vi "PFI-28000-System_Get Channels Per Card.vi"(8 "error in (no error)":errorcluster, 11 "PFI-28000-System in":refnum<class "PFI-28000-System.lvclass">) -> (0 "error out":errorcluster, 2 "Channels Per Card":i32, 3 "PFI-28000-System out":refnum<class "PFI-28000-System.lvclass">)   [LabVIEW 2017, in "PFI-28000-System.lvclass"]
uses:
  PFI-28000-System.lvclass
  Utilities/PFI-28000-Utils.lvlib
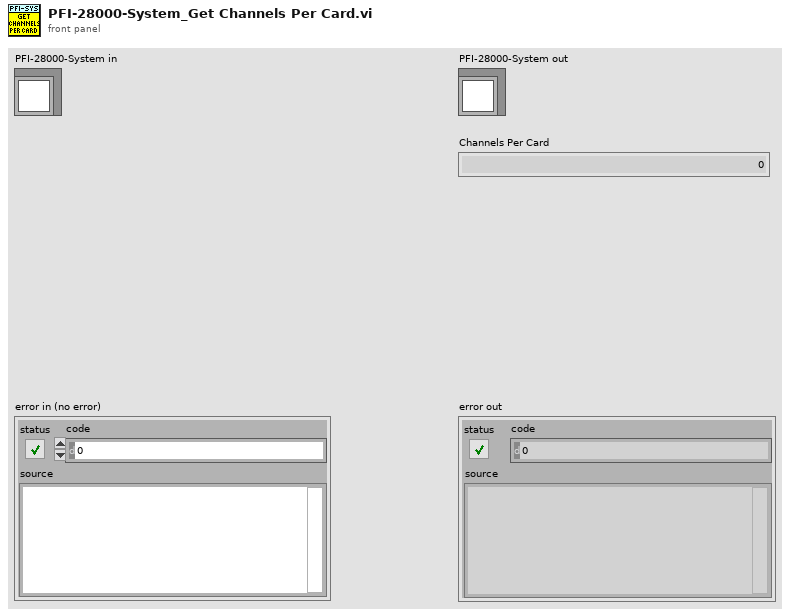
[diagram p1: front panel]
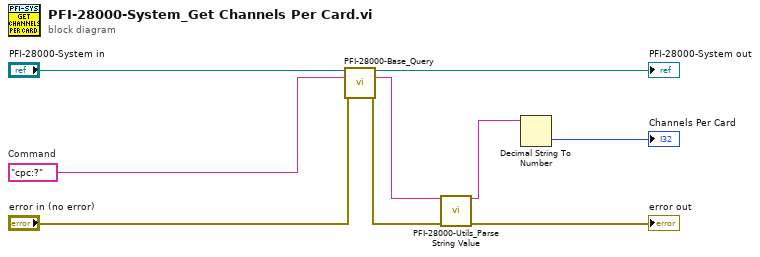
[diagram p0: block diagram]
diagram:
  w8 = "cpc:?"  # Command
  n1 = call-dynamic "PFI-28000-Base_Query.vi"("PFI-28000-Base in"="PFI-28000-System in", "Command"=w8, "error in (no error)"="error in (no error)") -> ("PFI-28000-Base out"=→"PFI-28000-System out":refnum<class "PFI-28000-System.lvclass">, "Response"=w4:string, "error out"=w6:errorcluster)  [unwired: 9 in, 1 out]
  n2 = call "PFI-28000-Utils_Parse String Value.vi"("String"=w4, "error in (no error)"=w6) -> ("String Value"=w2:string, "error out"=→"error out":errorcluster)  [unwired: 11 in, 1 out]
  n3 = Decimal String To Number(string=w2) -> (number=→"Channels Per Card":i32)  [unwired: 2 in, 1 out]
